vi "MB_SetActiveData_LoadedFromVI.vi"(7 "Layer Data":T1 {"Opacity" scale=0.0..100.0}, 8 "Error":errorcluster, 9 "Match?":bool, 10 "Match Index":i32, 11 "FakedArray":refnum<class "FakedArray.lvclass">) -> (0 "Error Out":errorcluster, 2 "Position Scrollbar Out":i32, 3 "FakedArray Out":refnum<class "FakedArray.lvclass">, 5 "Layer Data Out":T1={"LayerIcon"=bytes[3102], "LayerName"="", "Opacity"=100, "Visibility?"=TRUE} {"Opacity" scale=0.0..100.0})   [LabVIEW 2021, in "FakedArray.lvclass"]
uses:
  FakedArray.lvclass
  MB CORE/TypeDefs/Cluster_Layer Data.ctl
  MB CORE/TypeDefs/Cluster_Path&Icon.ctl
  FakedArray.lvclass/FakedArray.ctl
  vi.lib/LabVIEW Icon API/lv_icon/Controls/Pathes.ctl
  vi.lib/LabVIEW Icon API/lv_icon/lv_icon.lvlib
panel:
  in  "Filter":string="LabVIEW Icon API"
  out "Valid? Out":bool
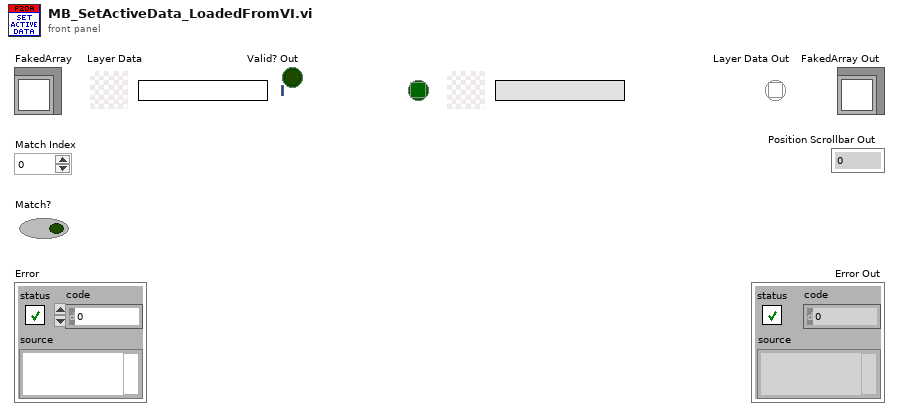
[diagram p1: front panel]
types:
  T1 = typedef "Cluster_Layer Data.ctl" = cluster{"LayerIcon":picture, "LayerName":string, "Opacity":u8, "Visibility?":bool}
  T2 = typedef "Cluster_Path&Icon.ctl" = cluster{"Rectangle":cluster{"left":i16, "top":i16, "right":i16, "bottom":i16}, "Path":path, "Image":picture, "Filter":string, "FileName":string}
  T3 = enum32{"Unknown Icon Source", "VI Icon", "Library Icon (any library type)", "Palette icon", "Icon from App Method"}
  T4 = typedef "Pathes.ctl" = enum16{"Root Path", "Icon Templates", "Icon Templates VI", "Icon Templates Lib", "Glyphs"}
  T5 = cluster{"left":i16, "top":i16, "right":i16, "bottom":i16}
  T6 = typedef "Who Invoked Icon Editor.ctl" = cluster{"Icon Editor Invoker Type":T7, "App Refnum of Invoker":refnum<vi>, "Qualified Name of Invoker":string, "Path to Invoker":path}
  T7 = typedef "Icon Editor Invoker Type.ctl" = enum32{"Unknown Icon Source", "VI Icon", "Library Icon (any library type)", "Palette icon", "Icon from App Method"}
  T8 = typedef "LabVIEW Icon Stored Information.ctl" = cluster{"Text Visible?":bool, "Text Opacity":u8, "Templ Visible?":bool, "Templ Opacity":u8, "Relative Path from 1 to 2":path, "Image":picture, "All User Layers":refnum<class "Layer.lvclass">[], "Body Text":T9}
  T9 = typedef "Cluster_BodyText.ctl" = cluster{"Line 1 text":string, "Line 2 text":string, "Line 3 text":string, "Line 4 text":string, "Line 1 color":u32, "Line 2 color":u32, "Line 3 color":u32, "Line 4 color":u32, "Body Text Spec":cluster{"Font":T10, "Alignment":T11, "Size":u8}, "Center text vertically":bool, "Capitalize Text":bool}
  T10 = typedef "Font.ctl" = string
  T11 = typedef "Alignment.ctl" = u16
  T12 = typedef "Cluster_INI Data.ctl" = cluster{"Show Layer Tab?":bool, "Show Terminals?":bool, "Text":cluster{"Font":T10, "Alignment":T11, "Size":T13}, "3rd party Templates":cluster{"Store 3rd party Templates?":bool, "Folder Name":string}, "Merge user layers on commit":bool, "Body Text":T9, "Fill Color":T14, "Edge Color":T14, "Tab":u16, "Tool":T15, "Disable Layers?":bool}
  T13 = typedef "Num_Font Size.ctl" = u8
  T14 = typedef "IEColor.ctl" = u32
  T15 = typedef "Cluster_Button Draw Tools.ctl" = enum32{"Pencil", "Line", "Dropper", "Fill", "Rectangle", "Filled Rectangle", "Ellipse", "Filled Ellipse", "Eraser", "Text", "Select", "Move"}
  T16 = typedef "imagedata.ctl" = cluster{"image type":i32, "image depth":i32, "image":u8[], "mask":u8[], "colors":u32[], "Rectangle":cluster{"left":i16, "top":i16, "right":i16, "bottom":i16}}
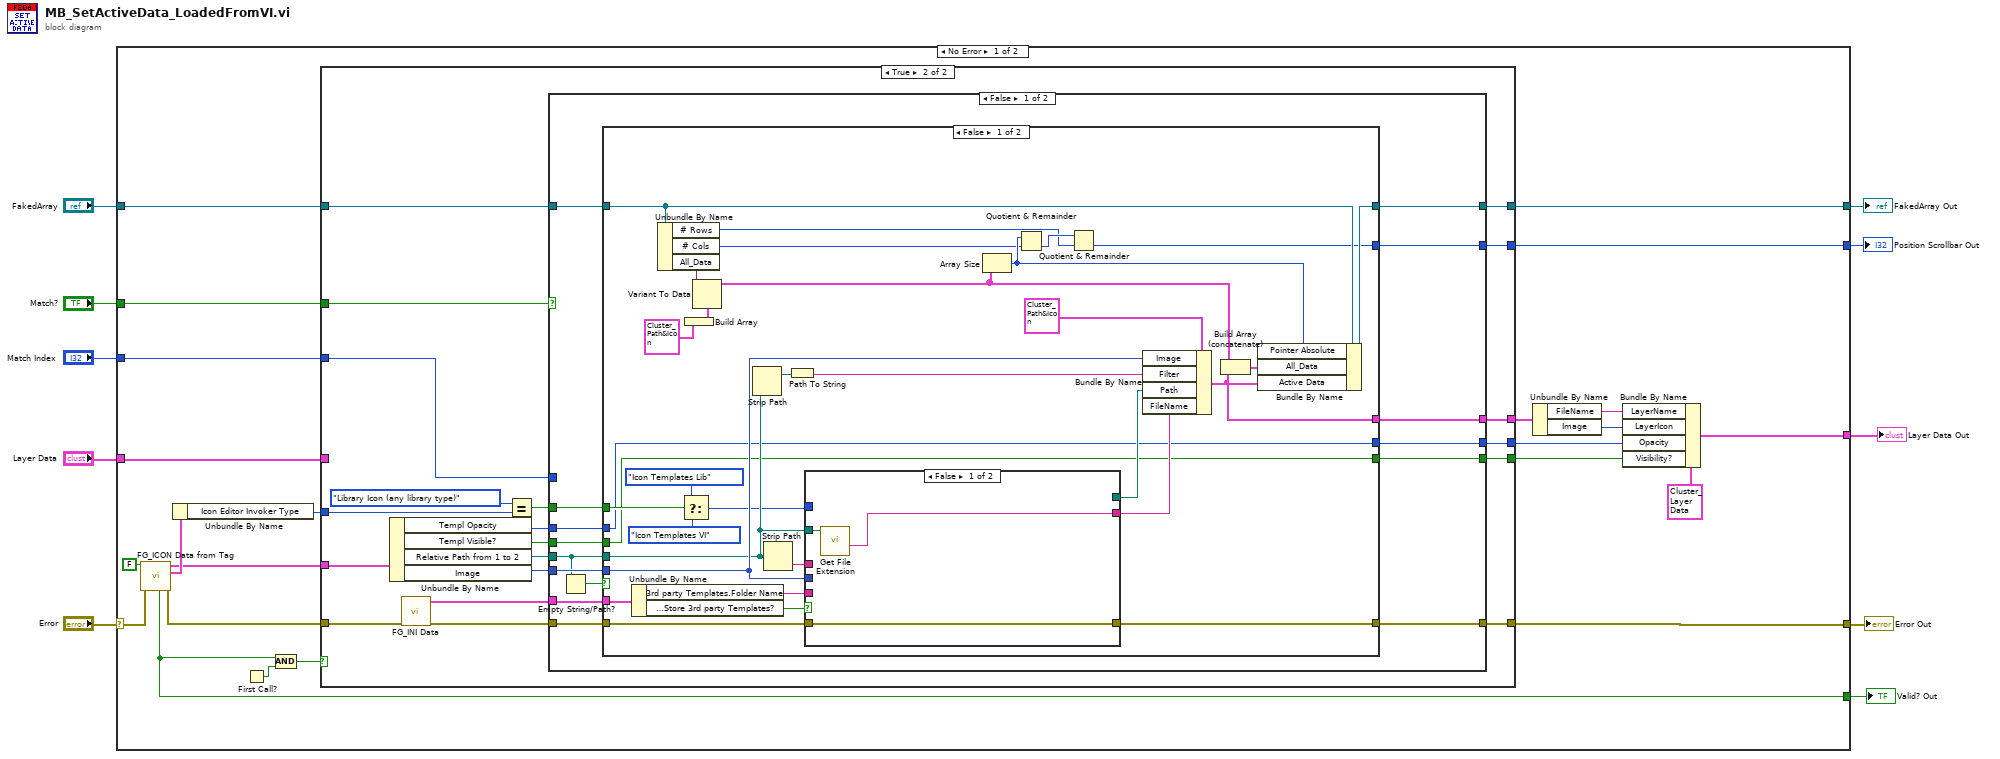
[diagram p0: block diagram]
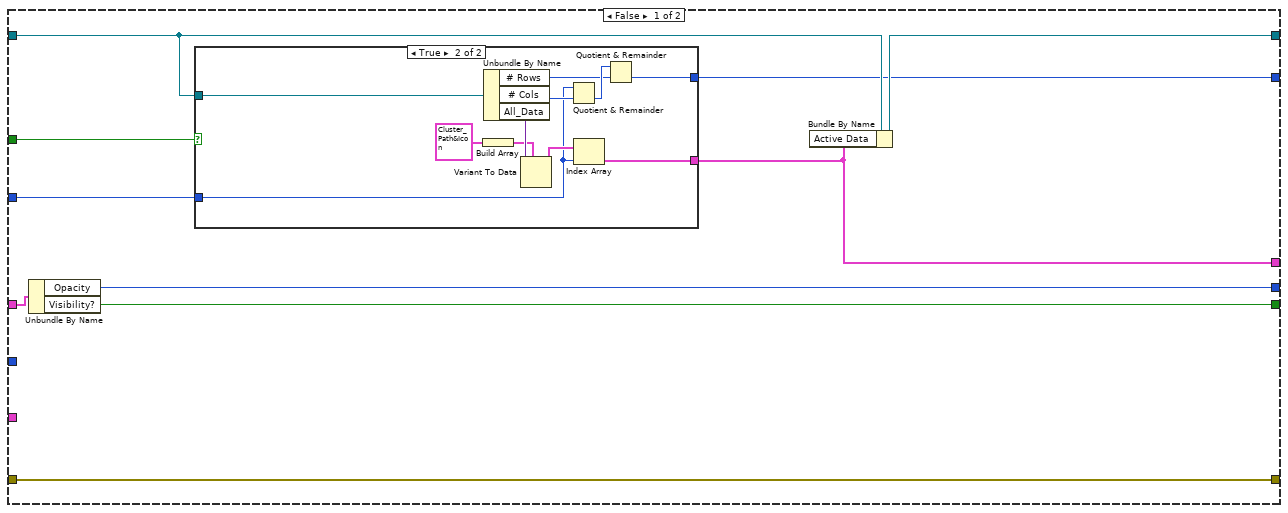
[diagram p2: hidden frame]
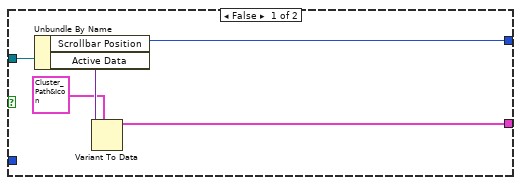
[diagram p3: hidden frame]
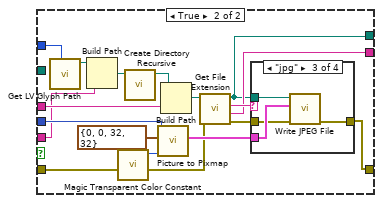
[diagram p4: hidden frame]
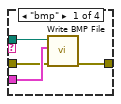
[diagram p5: hidden frame]
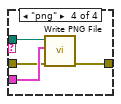
[diagram p7: hidden frame]
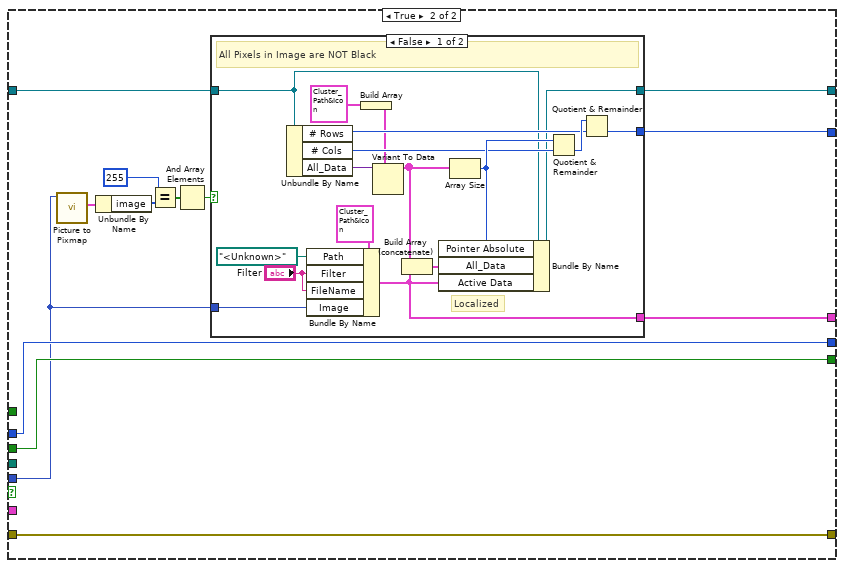
[diagram p8: hidden frame]
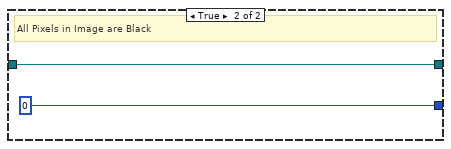
[diagram p9: hidden frame]
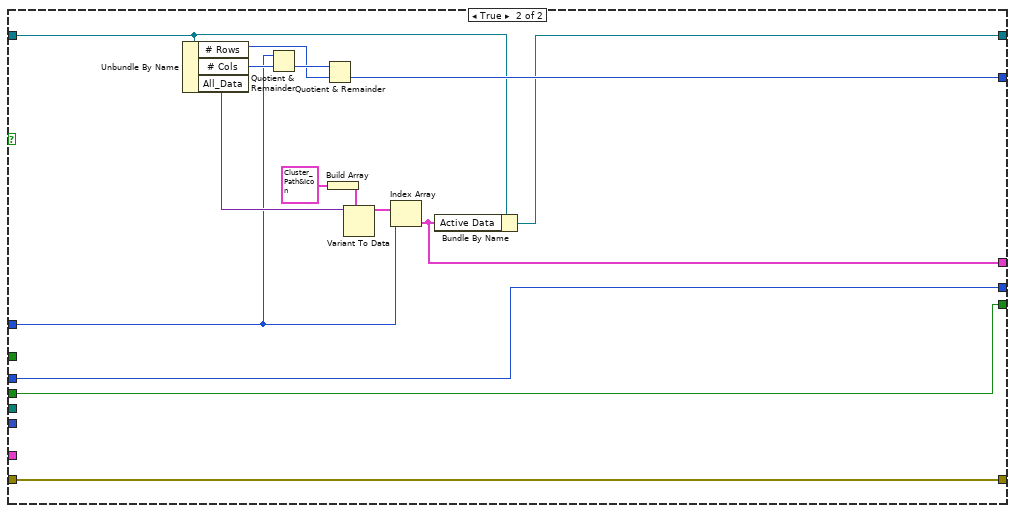
[diagram p10: hidden frame]
diagram:
  n1 = case shown="No Error" "Error" {
    selector: "Error" -> [w31 w208]
    tunnel: [w13 w208] -> w9
    tunnel: [w32 w207] -> w7
    tunnel: "FakedArray" -> [w33 w207]
    tunnel: "Match Index" -> [w28 _]
    tunnel: "Match?" -> [w29 _]
    tunnel: [w27 _] -> w4
    tunnel: [w21 _] -> w3
    tunnel: [w15 _] -> w2
    tunnel: "Layer Data" -> [w14 _]
    frame No Error {
      n2 = call "FG_ICON Data from Tag.vi"("Error"=w31, "Init? (F)"=FALSE) -> ("Error Out"=w30:errorcluster, "Invoked Data Out"=w26:T6, "Data Out"=w16:T8, "Valid? Out"=w21:bool)  [unwired: 1 in, 5 out]
      n3 = Unbundle By Name(w26) -> ("Icon Editor Invoker Type"=w11:T7)
      n4 = First Call?() -> (First Call?: T/F=w20:bool)
      n5 = And(x=w21, y=w20) -> (x .and. y?=w19:bool)
      n6 = case shown="True" w19 {
        tunnel: w33 -> [w42 w78]
        tunnel: [w41 w72] -> w32
        tunnel: w16 -> [_ w79]
        tunnel: w30 -> [w43 w75]
        tunnel: w29 -> [w37 w77]
        tunnel: w28 -> [w40 w74]
        tunnel: [w43 w73] -> w13
        tunnel: [w39 w71] -> w27
        tunnel: w11 -> [_ w67]
        tunnel: [w38 w64] -> w25
        tunnel: [w36 w61] -> w18
        tunnel: [w35 w60] -> w17
        tunnel: w14 -> [w34 _]
        frame False {
          n7 = Unbundle By Name(w34) -> ("Opacity"=w36:u8, "Visibility?"=w35:bool)
          n8 = case shown="True" w37 {
            tunnel: w42 -> [w48 w54]
            tunnel: w40 -> [_ w51]
            tunnel: [w47 w53] -> w39
            tunnel: [w45 w52] -> w38
            frame False {
              n9 = Unbundle By Name(w48) -> ("Scrollbar Position"=w47:i32, "Active Data"=w46:variant)
              n10 = Variant To Data(type=T2 {"Rectangle"={"left"=0, "top"=0, "right"=0, "bottom"=0}, "Path"=path "", "Image"=bytes[0], "Filter"="", "FileName"=""}, Variant=w46) -> (data=w45:T2)  [unwired: 1 in, 1 out]
            }
            frame True {
              n11 = Build Array(T2 {"Rectangle"={"left"=0, "top"=0, "right"=0, "bottom"=0}, "Path"=path "", "Image"=bytes[0], "Filter"="", "FileName"=""}) -> (w49:T2[])
              n12 = Unbundle By Name(w54) -> ("# Rows"=w57:i32, "# Cols"=w58:i32, "All_Data"=w56:variant)
              n13 = Variant To Data(type=w49, Variant=w56) -> (data=w55:T2[])  [unwired: 1 in, 1 out]
              n14 = Quotient & Remainder(x=w51, y=w58) -> (floor(x/y)=w59:i32)  [unwired: 1 out]
              n15 = Index Array(array=w55, index=w51) -> (element=w52:T2)
              n16 = Quotient & Remainder(x=w59, y=w57) -> (floor(x/y)=w53:i32)  [unwired: 1 out]
            }
          }
          n17 = Bundle By Name(cluster=w42, "Active Data"=w38) -> (w41:refnum<class "FakedArray.lvclass">)
        }
        frame True {
          n18 = Unbundle By Name(w79) -> ("Templ Opacity"=w62:u8, "Templ Visible?"=w63:bool, "Relative Path from 1 to 2"=w76:path, "Image"=w68:picture)
          n19 = call "FG_INI Data.vi"("Error"=w75) -> ("Error Out"=w69:errorcluster, "INI Data Out"=w70:T12)  [unwired: 9 out]
          n20 = Equal?(x=T3."Library Icon (any library type)", y=w67) -> (x = y?=w65:bool)
          n21 = case shown="False" w77 {
            tunnel: w78 -> [w90 w198]
            tunnel: w76 -> [w85 _]
            tunnel: w70 -> [w94 _]
            tunnel: w69 -> [w93 w206]
            tunnel: [w92 w206] -> w73
            tunnel: w74 -> [_ w196]
            tunnel: [w91 w197] -> w72
            tunnel: [w89 w202] -> w71
            tunnel: w68 -> [w88 _]
            tunnel: w65 -> [w87 _]
            tunnel: [w86 w194] -> w64
            tunnel: w63 -> [w83 w192]
            tunnel: w62 -> [w82 w193]
            tunnel: [w81 w193] -> w61
            tunnel: [w80 w192] -> w60
            frame False {
              n22 = Empty String/Path?(string/path=w85) -> (empty?=w84:bool)
              n23 = case shown="False" w84 {
                tunnel: w94 -> [w126 _]
                tunnel: w93 -> [w125 w172]
                tunnel: [w124 w172] -> w92
                tunnel: [w123 w166] -> w91
                tunnel: w90 -> [w122 w167]
                tunnel: [w114 w168] -> w89
                tunnel: w88 -> [w112 w165]
                tunnel: w87 -> [w111 _]
                tunnel: [w110 w169] -> w86
                tunnel: w85 -> [w109 _]
                tunnel: w83 -> [w98 w170]
                tunnel: w82 -> [w99 w171]
                tunnel: [w99 w171] -> w81
                tunnel: [w98 w170] -> w80
                frame False {
                  n24 = Unbundle By Name(w126) -> ("3rd party Templates.Folder Name"=w108:string, "3rd party Templates.Store 3rd party Templates?"=w106:bool)
                  n25 = Unbundle By Name(w122) -> ("# Rows"=w115:i32, "# Cols"=w117:i32, "All_Data"=w121:variant)
                  n26 = Select(t=Pathes."Icon Templates Lib" ("Path"), s=w111, f=Pathes."Icon Templates VI" ("Path")) -> (s? t:f=w101:T4)
                  n27 = Build Array(T2 {"Rectangle"={"left"=0, "top"=0, "right"=0, "bottom"=0}, "Path"=path "", "Image"=bytes[0], "Filter"="", "FileName"=""}) -> (w113:T2[])
                  n28 = Variant To Data(type=w113, Variant=w121) -> (data=w119:T2[])  [unwired: 1 in, 1 out]
                  n29 = Strip Path(path=w109) -> (stripped path=w100:path)  [unwired: 1 out]
                  n30 = Strip Path(path=w109) -> (name=w104:string)  [unwired: 1 out]
                  n31 = Path To String(path=w100) -> (string=w97:string)
                  n32 = case shown="False" w106 {
                    tunnel: w108 -> [_ w130]
                    tunnel: w125 -> [w128 w141]
                    tunnel: [w128 w139] -> w124
                    tunnel: [w129 w137] -> w107
                    tunnel: w112 -> [_ w136]
                    tunnel: [_ w134] -> w105
                    tunnel: w104 -> [_ w133]
                    tunnel: w109 -> [w127 _]
                    tunnel: w101 -> [_ w132]
                    frame False {
                      n33 = call <vilib>:"Get File Extension.vi"("file"=w127) -> ("filename without extension"=w129:string)  [unwired: 1 in, 9 out]
                    }
                    frame True {
                      n34 = call "Get LV Glyph Path.vi"("Path"=w132) -> ("Requested Path"=w146:path)  [unwired: 2 in, 8 out]
                      n35 = Build Path(base path=w146, name or relative path=w130) -> (appended path=w135:path)
                      n36 = call "Magic Transparent Color Constant.vi"() -> ("Magic transparent color constant"=w131:u32)  [unwired: 11 out]
                      n37 = call <vilib>:"Create Directory Recursive.vi"("directory"=w135) -> ("directory copy"=w144:path)  [unwired: 2 in, 4 out]
                      n38 = call <vilib>:"Picture to Pixmap.vi"("Background Color"=w131, "rect"=T5 {"left"=0, "top"=0, "right"=32, "bottom"=32}, "picture"=w136) -> ("image data"=w142:T16)  [unwired: 1 in, 7 out]
                      n39 = Build Path(base path=w144, name or relative path=w133) -> (appended path=w138:path)
                      n40 = call <vilib>:"Get File Extension.vi"("error in (no error)"=w141, "file"=w138) -> ("error out"=w140:errorcluster, "filename without extension"=w137:string, "lowercase file extension"=w143:string, "dup file"=w134:path)  [unwired: 6 out]
                      n41 = case shown="\"jpg\"" w143 {
                        tunnel: w134 -> [w150 _ w155 w159]
                        tunnel: w142 -> [w149 _ w154 w158]
                        tunnel: w140 -> [w148 w151 w153 w157]
                        tunnel: [w147 w151 w152 w156] -> w139
                        frame "bmp" {
                          n42 = call <vilib>:"Write BMP File.vi"("error in (no error)"=w148, "image data"=w149, "path to BMP file"=w150) -> ("error out"=w147:errorcluster)  [unwired: 8 out]
                        }
                        frame Default {
                        }
                        frame "jpg" {
                          n43 = call <vilib>:"Write JPEG File.vi"("error in (no error)"=w153, "image data"=w154, "path to JPEG file"=w155) -> ("error out"=w152:errorcluster)  [unwired: 8 out]
                        }
                        frame "png" {
                          n44 = call <vilib>:"Write PNG File.vi"("error in (no error)"=w157, "image data"=w158, "path to PNG file"=w159) -> ("error out"=w156:errorcluster)  [unwired: 8 out]
                        }
                      }
                    }
                  }
                  n45 = Array Size(array=w119) -> (size(s)=w118:i32)
                  n46 = Quotient & Remainder(x=w118, y=w117) -> (floor(x/y)=w116:i32)  [unwired: 1 out]
                  n47 = Quotient & Remainder(x=w116, y=w115) -> (floor(x/y)=w114:i32)  [unwired: 1 out]
                  n48 = Bundle By Name(cluster=T2 {"Rectangle"={"left"=0, "top"=0, "right"=0, "bottom"=0}, "Path"=path "", "Image"=bytes[0], "Filter"="", "FileName"=""}, "Image"=w112, "Filter"=w97, "Path"=w105, "FileName"=w107) -> (w110:T2)
                  n49 = Build Array (concatenate)(w119, w110) -> (w120:T2[])
                  n50 = Bundle By Name(cluster=w122, "Pointer Absolute"=w118, "All_Data"=w120, "Active Data"=w110) -> (w123:refnum<class "FakedArray.lvclass">)
                }
                frame True {
                  n51 = call <vilib>:"Picture to Pixmap.vi"("picture"=w165) -> ("image data"=w164:T16)  [unwired: 9 in, 1 out]
                  n52 = Unbundle By Name(w164) -> ("image"=w163:u8[])
                  n53 = Equal?(x=u8 255, y=w163) -> (x = y?=w161:bool[])
                  n54 = And Array Elements(Boolean array=w161) -> (logical AND=w160:bool)
                  n55 = case shown="False" w160 {
                    tunnel: [w179 _] -> w169
                    tunnel: [w178 0] -> w168
                    tunnel: w167 -> [w173 w191]
                    tunnel: [w177 w191] -> w166
                    tunnel: w165 -> [w176 _]
                    frame False {
                      # "Localized"
                      # "All Pixels in Image are NOT Black"
                      n56 = Unbundle By Name(w173) -> ("# Rows"=w182:i32, "# Cols"=w184:i32, "All_Data"=w188:variant)
                      n57 = Bundle By Name(cluster=T2 {"Rectangle"={"left"=0, "top"=0, "right"=0, "bottom"=0}, "Path"=path "", "Image"=bytes[0], "Filter"="", "FileName"=""}, "Path"=path "<Unknown>", "Filter"="Filter", "FileName"="Filter", "Image"=w176) -> (w179:T2)
                      n58 = Build Array(T2 {"Rectangle"={"left"=0, "top"=0, "right"=0, "bottom"=0}, "Path"=path "", "Image"=bytes[0], "Filter"="", "FileName"=""}) -> (w181:T2[])
                      n59 = Variant To Data(type=w181, Variant=w188) -> (data=w186:T2[])  [unwired: 1 in, 1 out]
                      n60 = Build Array (concatenate)(w186, w179) -> (w187:T2[])
                      n61 = Array Size(array=w186) -> (size(s)=w185:i32)
                      n62 = Bundle By Name(cluster=w173, "Pointer Absolute"=w185, "All_Data"=w187, "Active Data"=w179) -> (w177:refnum<class "FakedArray.lvclass">)
                      n63 = Quotient & Remainder(x=w185, y=w184) -> (floor(x/y)=w183:i32)  [unwired: 1 out]
                      n64 = Quotient & Remainder(x=w183, y=w182) -> (floor(x/y)=w178:i32)  [unwired: 1 out]
                    }
                    frame True {
                      # "All Pixels in Image are Black"
                    }
                  }
                }
              }
            }
            frame True {
              n65 = Unbundle By Name(w198) -> ("# Rows"=w203:i32, "# Cols"=w204:i32, "All_Data"=w199:variant)
              n66 = Quotient & Remainder(x=w196, y=w204) -> (floor(x/y)=w205:i32)  [unwired: 1 out]
              n67 = Quotient & Remainder(x=w205, y=w203) -> (floor(x/y)=w202:i32)  [unwired: 1 out]
              n68 = Build Array(T2 {"Rectangle"={"left"=0, "top"=0, "right"=0, "bottom"=0}, "Path"=path "", "Image"=bytes[0], "Filter"="", "FileName"=""}) -> (w200:T2[])
              n69 = Variant To Data(type=w200, Variant=w199) -> (data=w195:T2[])  [unwired: 1 in, 1 out]
              n70 = Index Array(array=w195, index=w196) -> (element=w194:T2)
              n71 = Bundle By Name(cluster=w198, "Active Data"=w194) -> (w197:refnum<class "FakedArray.lvclass">)
            }
          }
        }
      }
      n72 = Unbundle By Name(w25) -> ("FileName"=w23:string, "Image"=w22:picture)
      n73 = Bundle By Name(cluster=T1 {"LayerIcon"=bytes[0], "LayerName"="", "Opacity"=0, "Visibility?"=FALSE}, "LayerName"=w23, "LayerIcon"=w22, "Opacity"=w18, "Visibility?"=w17) -> (w15:T1)
    }
    frame Error {
    }
  }
  "Error Out" <- w9
  "FakedArray Out" <- w7
  "Position Scrollbar Out" <- w4
  "Valid? Out" <- w3
  "Layer Data Out" <- w2
